vi "Write FWHM Gaussfit 2.vi"(8 "error in (no error)":errorcluster, 10 "FWHM Gaussfit":refnum<vi>, 11 "Analyze Results SHG-AK in":refnum<class "Analyze Results SHG-AK.lvclass">) -> (0 "error out":errorcluster, 3 "Analyze Results SHG-AK out":refnum<class "Analyze Results SHG-AK.lvclass">)   [LabVIEW 2014, in "Analyze Results SHG-AK.lvclass"]
uses:
  Analyze Results SHG-AK.lvclass
  Analyze Results SHG-AK.lvclass/Analyze Results SHG-AK.ctl
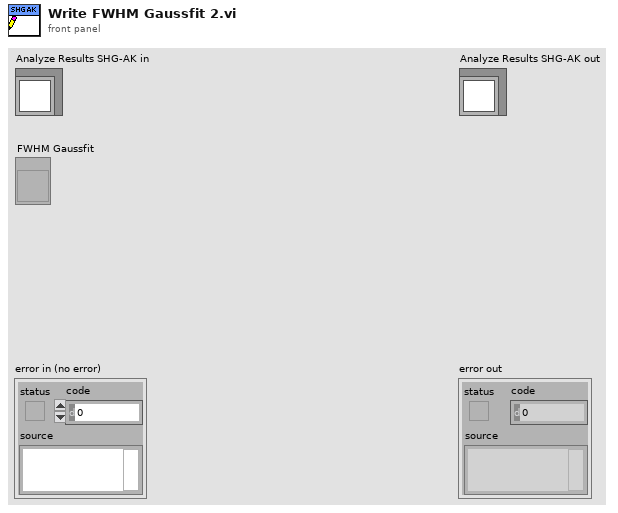
[diagram p1: front panel]
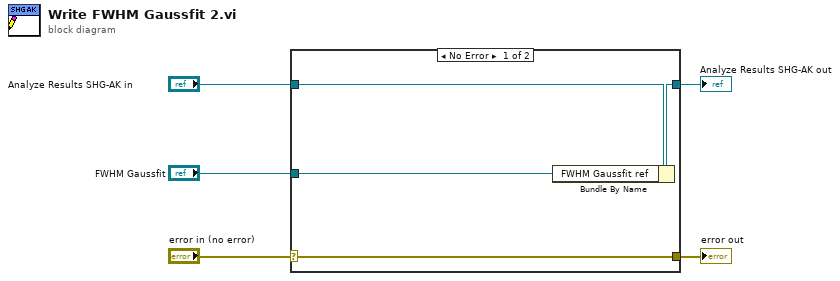
[diagram p0: block diagram]
diagram:
  n1 = case shown="No Error" "error in (no error)" {
    selector: "error in (no error)" -> [w9 w10]
    tunnel: [w9 w10] -> w4
    tunnel: [w7 w11] -> w2
    tunnel: "Analyze Results SHG-AK in" -> [w8 w11]
    tunnel: "FWHM Gaussfit" -> [w6 _]
    frame No Error {
      n2 = Bundle By Name(cluster=w8, "FWHM Gaussfit ref"=w6) -> (w7:refnum<class "Analyze Results SHG-AK.lvclass">)
    }
    frame Error {
    }
  }
  "error out" <- w4
  "Analyze Results SHG-AK out" <- w2
